vi "Pythagoras.vi"(1 "A":dbl, 2 "B":dbl) -> (0 "C":dbl format="%#.2g")   [LabVIEW 2020]
doc: "Liczy długość przeciwprostokątnej w oparciu o twierdzenie Pitagorasa"
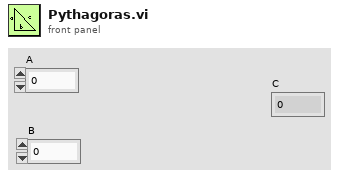
[diagram p1: front panel]
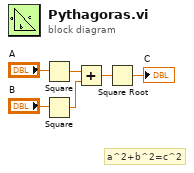
[diagram p0: block diagram]
diagram:
  # "a^2+b^2=c^2"
  n1 = Square(x="A") -> (x^2=w4:dbl)
  n2 = Square(x="B") -> (x^2=w3:dbl)
  n3 = Add(x=w4, y=w3) -> (x+y=w2:dbl)
  n4 = Square Root(x=w2) -> (sqrt(x)=→"C":dbl)
